vi "Supported Smart Syntax Representation.vi"(0 "Message Popup in":refnum<class "SMU.lvclass">, 11 "error in (no error)":errorcluster) -> (4 "Message Popup out":refnum<class "SMU.lvclass">, 6 "Smart Syntax Representation List":string[](array[string]), 15 "error out":errorcluster)   [LabVIEW 2016, in "SMU.lvclass"]
uses:
  SMU.lvclass
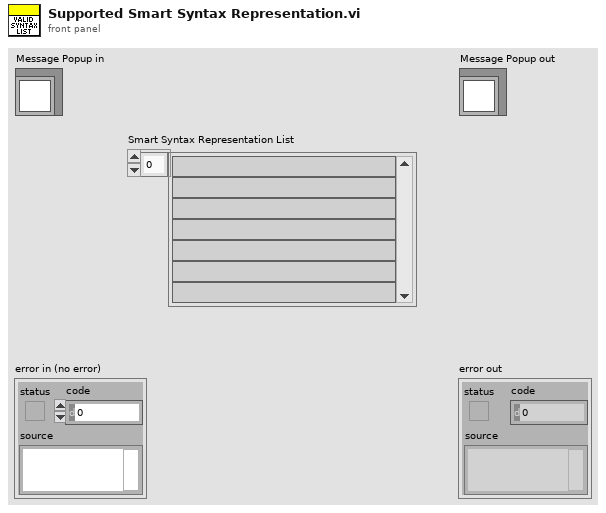
[diagram p1: front panel]
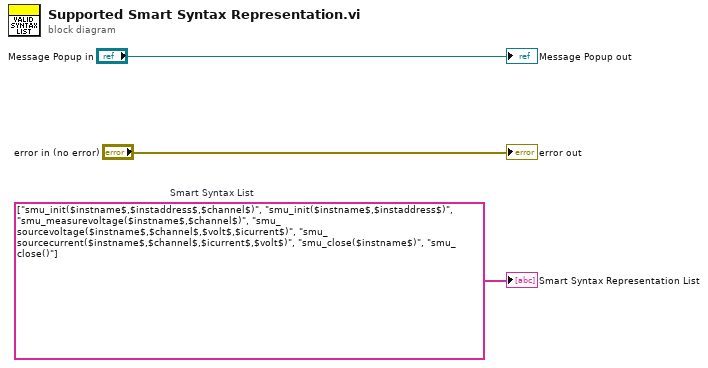
[diagram p0: block diagram]
diagram:
  w1 = string[] ["smu_init($instname$,$instaddress$,$channel$)", "smu_init($instname$,$instaddress$)", "smu_measurevoltage($instname$,$channel$)", "smu_sourcevoltage($instname$,$channel$,$volt$,$icurrent$)", "smu_sourcecurrent($instname$,$channel$,$icurrent$,$volt$)", "smu_close($instname$)", "smu_close()"]  # Smart Syntax List
  "error out" <- "error in (no error)"
  "Message Popup out" <- "Message Popup in"
  "Smart Syntax Representation List" <- w1
